vi "Persistent (No Objects).vi"(7 "Field monitor ref":refnum<vi>, 8 "error in (no error)":errorcluster, 10 "Go to persistent mode?":bool, 11 "Cluster In":T4={"Field"=0.0, "Rate"=0.0, "Status"={"Sweeping"=FALSE, "Clamped"=FALSE, "Hold"=FALSE, "At Rest"=FALSE, "Quench"=FALSE, "Persistent Mode"=FALSE, "Switch Heater"=FALSE}, "ILM Shut Down?"=FALSE, "IO Info"={"Address"={"Com Port"=1, "ISOBUS Address"=2, "GPIB Address"=24, "Communication"=enum."ISOBUS"}, "Version"=enum."IPS"}, "IO Info (Level Meter)"={"Address"={"Com Port"=1, "ISOBUS Address"=5, "GPIB Address"=24, "Communication"=enum."ISOBUS"}, "ILM Name"="", "Display Channel"=[]}, "Training?"=FALSE, "Training Field and Speed Cluster"={"Training Field"=[0.0, 4.108, 5.78, 8.001], "Training Speed"=[0.0057, 0.0022833333333333334, 0.0011333333333333334, 0.0011333333333333334]}}) -> (0 "error out":errorcluster, 3 "Cluster Out":T4={"Field"=0.0, "Rate"=0.0, "Status"={"Sweeping"=FALSE, "Clamped"=FALSE, "Hold"=FALSE, "At Rest"=FALSE, "Quench"=FALSE, "Persistent Mode"=FALSE, "Switch Heater"=FALSE}, "ILM Shut Down?"=FALSE, "IO Info"={"Address"={"Com Port"=1, "ISOBUS Address"=2, "GPIB Address"=24, "Communication"=enum."ISOBUS"}, "Version"=enum."IPS"}, "IO Info (Level Meter)"={"Address"={"Com Port"=1, "ISOBUS Address"=5, "GPIB Address"=24, "Communication"=enum."ISOBUS"}, "ILM Name"="", "Display Channel"=[]}, "Training?"=FALSE, "Training Field and Speed Cluster"={"Training Field"=[0.0, 4.108, 5.78, 8.001], "Training Speed"=[0.0057, 0.0022833333333333334, 0.0011333333333333334, 0.0011333333333333334]}})   [LabVIEW 2012]
doc: "Persistent mode closes the switch and turns off the power supply. The superconducting electromagnet will then remain energized indefinitely.\n\nTo leave persistent mode, you must first ramp up the power supply to match the energized magnet, then open the switch. \n\nA current mismatch is dangerous! The magnet will forbid opening the switch unless the power supply matches the energized magnet."
uses:
  Magnet status.ctl
  Oxford/PSSUBS.LLB/PSIO.ctl
  Oxford/BUSGEN.LLB/OxfordAddress.ctl
  Global/Relative Sound Files.vi
  Power Supply.lvclass
panel:
  out "Power Supply Output \"Field\"":dbl[unit]
  out "SHon?":bool caption="Switch Heater"
  out "persis?":bool caption="Persistent"
  out "title":string
  out "Actual Field":dbl[unit]
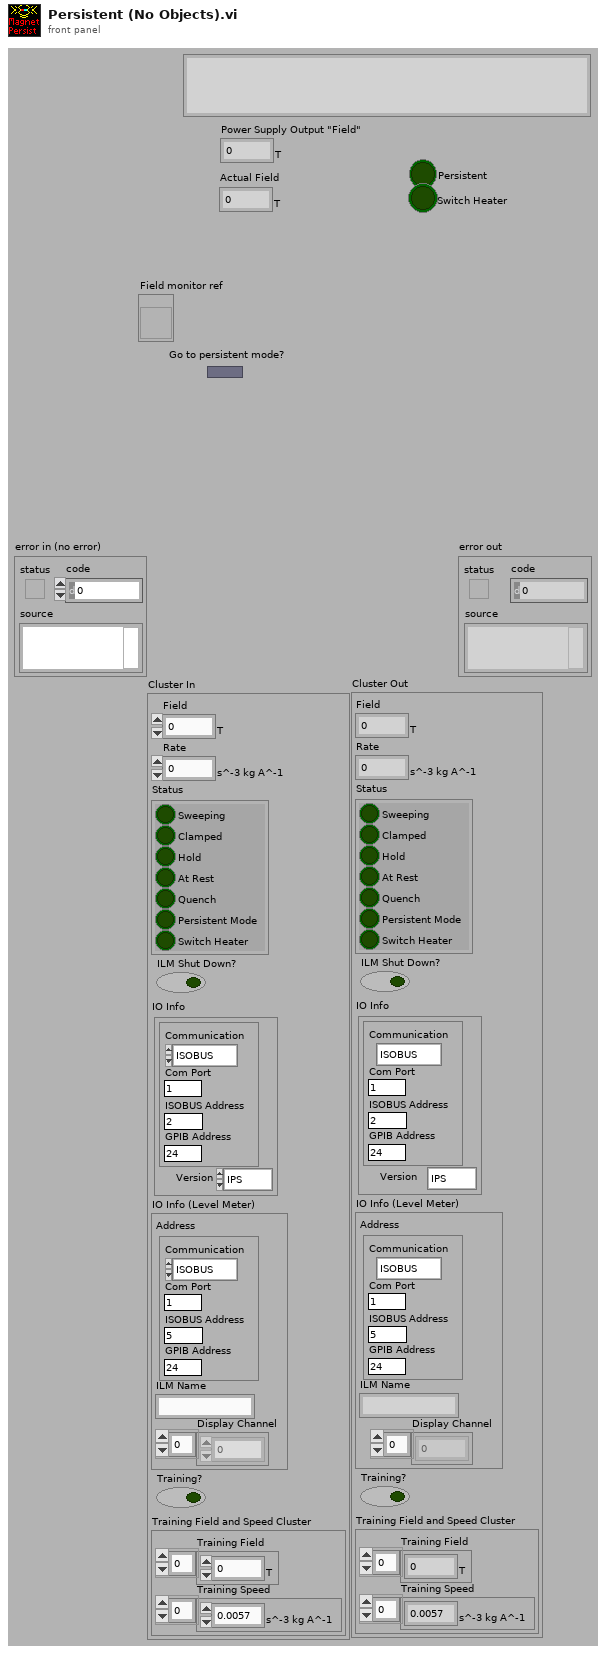
[diagram p1: front panel]
types:
  T1 = typedef "Power Supply.lvclass/Magnet status.ctl" = cluster{"Sweeping":bool, "Clamped":bool, "Hold":bool, "At Rest":bool, "Quench":bool, "Persistent Mode":bool, "Switch Heater":bool}
  T2 = typedef "PSIO.ctl" = cluster{"Address":T3, "Version":enum16{"PS", "IPS"}}
  T3 = typedef "OxfordAddress.ctl" = cluster{"Com Port":i32, "ISOBUS Address":i32, "GPIB Address":i16, "Communication":enum16{"RS232", "ISOBUS", "GPIB", "Gateway"}}
  T4 = cluster{"Field":dbl[unit], "Rate":dbl[unit], "Status":T1, "ILM Shut Down?":bool, "IO Info":T2, "IO Info (Level Meter)":cluster{"Address":T3, "ILM Name":string, "Display Channel":i32[]}, "Training?":bool, "Training Field and Speed Cluster":cluster{"Training Field":dbl[unit][], "Training Speed":dbl[unit][]}}
  T5 = typedef "Power Supply.lvclass/Switch Heater Status.ctl" = enum16{"Off (at zero)", "On", "Off (at field)", "Other"}
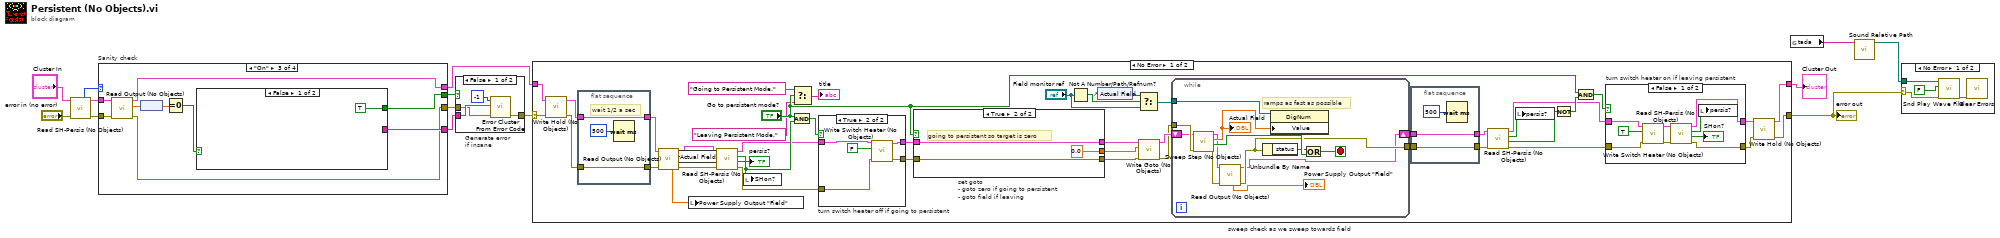
[diagram p0: block diagram]
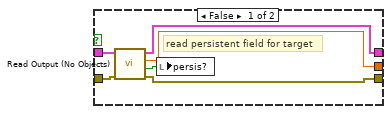
[diagram p3: hidden frame]
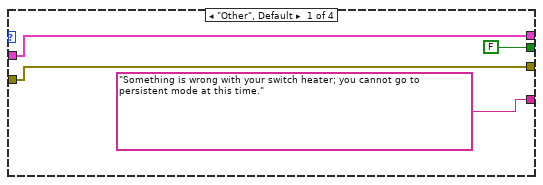
[diagram p7: hidden frame]
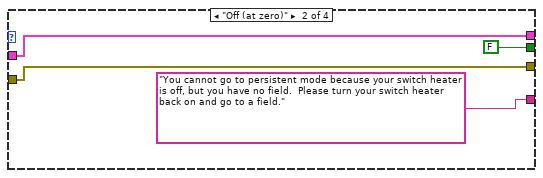
[diagram p8: hidden frame]
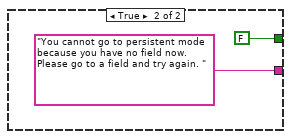
[diagram p9: hidden frame]
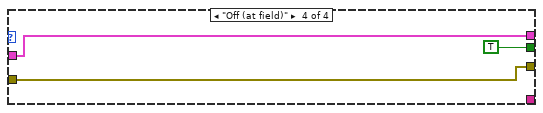
[diagram p10: hidden frame]
diagram:
  n1 = call "Read SH-Persis (No Objects).vi"("error in (no error)"="error in (no error)", "Cluster In"="Cluster In") -> ("error out"=w8:errorcluster, "Cluster Out"=w10:T4, "SHstatus"=w13:T5)  [unwired: 4 in, 3 out]
  n2 = case "Sanity check" shown="\"On\"" w13 {
    tunnel: [FALSE FALSE w31 TRUE] -> w12
    tunnel: ["Something is wrong with your switch heater; you cannot go to persistent mode at this time." "You cannot go to persistent mode because your switch heater is off, but you have no field.  Please turn your switch heater back on and go to a field." w28 _] -> w11
    tunnel: w10 -> [w16 w20 w23 w36]
    tunnel: [w16 w20 w27 w36] -> w14
    tunnel: [w15 w19 w26 w35] -> w9
    tunnel: w8 -> [w15 w19 w25 w35]
    frame "Other", Default {
    }
    frame "Off (at zero)" {
    }
    frame "On" {
      n3 = call "Read Output (No Objects).vi"("error in (no error)"=w25, "Cluster In"=w23) -> ("error out"=w26:errorcluster, "Field"=w30:dbl[unit], "Cluster Out"=w27:T4)  [unwired: 5 in, 2 out]
      n4 = node(w30) -> (w24:dbl)
      n5 = Equal To 0?(x=w24) -> (x = 0?=w29:bool)
      n6 = case shown="False" w29 {
        tunnel: [TRUE FALSE] -> w31
        tunnel: [_ "You cannot go to persistent mode because you have no field now.  Please go to a field and try again. "] -> w28
        frame False {
        }
        frame True {
        }
      }
    }
    frame "Off (at field)" {
    }
  }
  n7 = case "Generate error\nif insane" shown="False" w12 {
    tunnel: w11 -> [w40 _]
    tunnel: [w39 w42] -> w6
    tunnel: w9 -> [w38 w42]
    frame False {
      n8 = call <vilib>:"Error Cluster From Error Code.vi"("error in (no error)"=w38, "error message (\"\")"=w40, "error code (0)"=-1) -> ("error out"=w39:errorcluster)  [unwired: 6 in]
    }
    frame True {
    }
  }
  n9 = case shown="No Error" w6 {
    selector: w6 -> [w54 w133]
    tunnel: [w85 w132] -> w1
    tunnel: [w84 w133] -> w5
    tunnel: w14 -> [w49 w132]
    frame No Error {
      n10 = call "Write Hold (No Objects).vi"("error in (no error)"=w54, "Cluster In"=w49) -> ("error out"=w55:errorcluster, "Cluster Out"=w57:T4)  [unwired: 8 in]
      n11 = flat-sequence {
        tunnel: w57 -> [w89]
        tunnel: [w89] -> w48
        tunnel: [w88] -> w56
        tunnel: w55 -> [w88]
        frame #0 {
          # "wait 1/2 a sec"
          n12 = Wait (ms)(milliseconds to wait=500) -> ()  [unwired: 1 out]
        }
      }
      n13 = call "Read Output (No Objects).vi"("error in (no error)"=w56, "Cluster In"=w48) -> ("error out"=w64:errorcluster, "Field"=w58:dbl[unit], "Cluster Out"=w47:T4, "Power supply \"field\""=w43:dbl[unit])  [unwired: 5 in, 1 out]
      n14 = local write "Actual Field"(w58) -> ()
      n15 = local write "Power Supply Output \"Field\""(w43) -> ()
      n16 = call "Read SH-Persis (No Objects).vi"("error in (no error)"=w64, "Cluster In"=w47) -> ("error out"=w62:errorcluster, "SHon?"=w66:bool, "pers?"=→"persis?":bool, "Cluster Out"=w63:T4)  [unwired: 4 in, 2 out]
      n17 = local write "SHon?"(w66) -> ()
      n18 = And(x="Go to persistent mode?", y=w66) -> (x .and. y?=w67:bool)
      n19 = Select(t="Going to Persistent Mode.", s="Go to persistent mode?", f="Leaving Persistent Mode.") -> (s? t:f=→"title":string)
      n20 = case "turn switch heater off if going to persistent" shown="True" w67 {
        tunnel: [w91 w95] -> w70
        tunnel: w63 -> [w91 w92]
        tunnel: w62 -> [w90 w94]
        tunnel: [w90 w93] -> w69
        frame False {
        }
        frame True {
          n21 = call "Write Switch Heater (No Objects).vi"("error in (no error)"=w94, "Turn SH On?"=FALSE, "Cluster In"=w92) -> ("error out"=w93:errorcluster, "Cluster Out"=w95:T4)  [unwired: 7 in]
        }
      }
      n22 = case "set goto\n- goto zero if going to persistent\n- goto field if leaving" shown="True" "Go to persistent mode?" {
        tunnel: [w101 dbl[unit] 0.0 ("Field")] -> w71
        tunnel: [w100 w104] -> w46
        tunnel: w70 -> [w97 w104]
        tunnel: w69 -> [w99 w103]
        tunnel: [w98 w103] -> w68
        frame False {
          # "read persistent field for target"
          n23 = call "Read Output (No Objects).vi"("error in (no error)"=w99, "Cluster In"=w97) -> ("error out"=w98:errorcluster, "persistent?"=w102:bool, "Field"=w101:dbl[unit], "Cluster Out"=w100:T4)  [unwired: 5 in, 1 out]
          n24 = local write "persis?"(w102) -> ()
        }
        frame True {
          # "going to persistent so target is zero"
        }
      }
      n25 = Not A Number/Path/Refnum?(number/path/refnum="Field monitor ref") -> (NaN/Path/Refnum?=w53:bool)
      n26 = control-ref of="Actual Field"() -> (w52:refnum<vi>)
      n27 = Select(t=w52, s=w53, f="Field monitor ref") -> (s? t:f=w50:refnum<vi>)
      n28 = call "Write Goto (No Objects).vi"("error in (no error)"=w68, "Target"=w71, "Cluster In"=w46) -> ("error out"=w72:errorcluster, "Cluster Out"=w73:T4)  [unwired: 7 in]
      n29 = while "sweep check as we sweep towards field" {
        shift-right: [w107] -> w75
        shift-left: w73 -> [w111]
        tunnel: [w108] -> w74
        tunnel: w72 -> [w116]
        tunnel: w50 -> [w115]
        stop <- w113 stop-if-true
        # "ramps as fast as possible"
        n30 = call "Sweep Step (No Objects).vi"("error in (no error)"=w116, "Cluster In"=w111) -> ("error out"=w109:errorcluster, "Done?"=w117:bool, "field"=w114:dbl[unit], "Cluster Out"=w110:T4)  [unwired: 5 in, 1 out]
        "Actual Field" <- w114
        n31 = call "Read Output (No Objects).vi"("error in (no error)"=w109, "Cluster In"=w110) -> ("error out"=w108:errorcluster, "Cluster Out"=w107:T4, "Power supply \"field\""=→"Power Supply Output \"Field\"":dbl[unit])  [unwired: 5 in, 2 out]
        n32 = Unbundle By Name(w108) -> ("status"=w112:bool)
        n33 = property on="Property Node" class="DigNum"(reference=w115, "Value"=w114) -> ()  [unwired: 1 in, 2 out]
        n34 = Or(x=w112, y=w117) -> (x .or. y?=w113:bool)
      }
      n35 = flat-sequence {
        tunnel: w75 -> [w119]
        tunnel: [w119] -> w45
        tunnel: w74 -> [w118]
        tunnel: [w118] -> w78
        frame #0 {
          n36 = Wait (ms)(milliseconds to wait=500) -> ()  [unwired: 1 out]
        }
      }
      n37 = call "Read SH-Persis (No Objects).vi"("error in (no error)"=w78, "Cluster In"=w45) -> ("error out"=w77:errorcluster, "SHon?"=w80:bool, "pers?"=w79:bool, "Cluster Out"=w76:T4)  [unwired: 4 in, 2 out]
      n38 = local write "persis?"(w79) -> ()
      n39 = Not(x=w80) -> (.not. x?=w81:bool)
      n40 = And(x="Go to persistent mode?", y=w81) -> (x .and. y?=w82:bool)
      n41 = case "turn switch heater on if leaving persistent" shown="False" w82 {
        tunnel: [w126 w130] -> w83
        tunnel: w77 -> [w129 w130]
        tunnel: w76 -> [w122 w131]
        tunnel: [w123 w131] -> w44
        frame False {
          n42 = call "Write Switch Heater (No Objects).vi"("error in (no error)"=w129, "Turn SH On?"=TRUE, "Cluster In"=w122) -> ("error out"=w127:errorcluster, "Cluster Out"=w121:T4)  [unwired: 7 in]
          n43 = call "Read SH-Persis (No Objects).vi"("error in (no error)"=w127, "Cluster In"=w121) -> ("error out"=w126:errorcluster, "SHon?"=→"SHon?":bool, "pers?"=w124:bool, "Cluster Out"=w123:T4)  [unwired: 4 in, 2 out]
          n44 = local write "persis?"(w124) -> ()
        }
        frame True {
        }
      }
      n45 = call "Write Hold (No Objects).vi"("error in (no error)"=w83, "Cluster In"=w44) -> ("error out"=w84:errorcluster, "Cluster Out"=w85:T4)  [unwired: 8 in]
    }
    frame Error {
    }
  }
  "error out" <- w5
  "Cluster Out" <- w1
  n46 = global read "Relative Sound Files.vi" "tada"() -> (w4:string)
  n47 = call "Sound Relative Path.vi"("Sound"=w4) -> ("Relative Path"=w3:path)  [unwired: 10 in]
  n48 = case shown="No Error" w5 {
    selector: w5 -> [w134 _]
    tunnel: w3 -> [w137 _]
    frame No Error {
      n49 = call <vilib>:"Snd Play Wave File.vi"("error in (no error)"=w134, "wait until finish (T)"=FALSE, "wave file path"=w137) -> ("error out"=w135:errorcluster)  [unwired: 8 out]
      n50 = call <vilib>:"Clear Errors.vi"("error in (no error)"=w135) -> ()  [unwired: 6 in, 1 out]
    }
    frame Error {
    }
  }
